vi "Create WebProxy.vi"(4 "BypassProxyOnLocal":bool, 5 "WebProxy":refnum<class "WebProxy_NET.lvclass">, 6 "UseDefaultCredentials [T]":bool, 8 "Error In":errorcluster, 10 "Port (443)":i32=443, 11 "Host":string) -> (0 "Error Out":errorcluster, 3 "WebProxy Out":refnum<class "WebProxy_NET.lvclass">)   [LabVIEW 2024, in "HttpClient_NET.lvlib" / "WebProxy_NET.lvclass"]
doc: "<b> </b> <b> </b>\nHttpClient_NET\nJustin Young - Viviota\nCopyright (c) 2021\nLicense: BSD"
uses:
  WebProxy_NET.lvclass
  WebProxy_NET.lvclass/WebProxy_NET.ctl
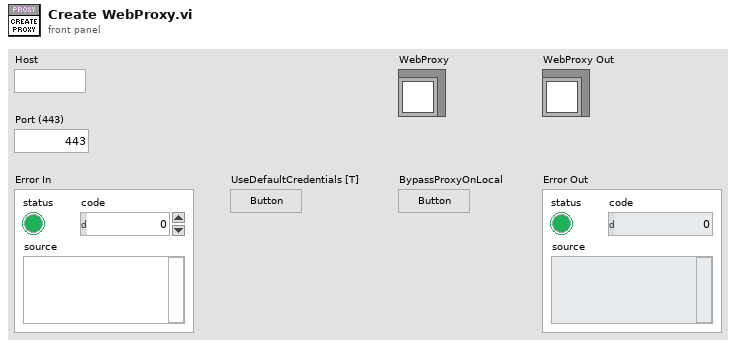
[diagram p1: front panel]
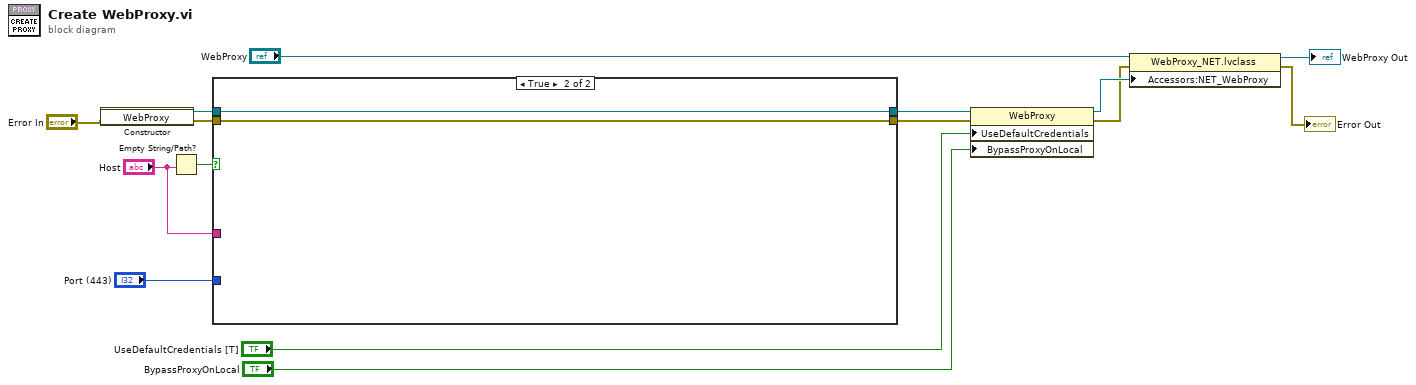
[diagram p0: block diagram]
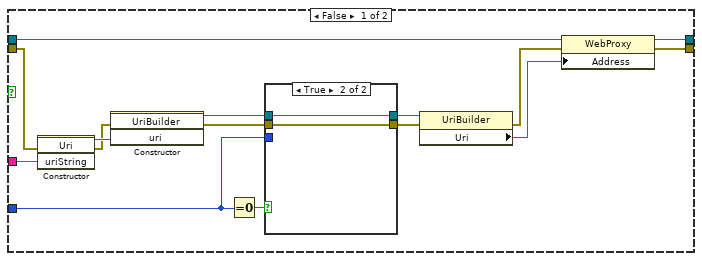
[diagram p2: hidden frame]
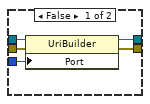
[diagram p3: hidden frame]
diagram:
  n1 = constructor class="WebProxy"(error in="Error In") -> (reference out=w8:refnum<k24>, error out=w15:errorcluster)  [unwired: 2 in, 1 out]
  n2 = Empty String/Path?(string/path="Host") -> (empty?=w4:bool)
  n3 = case shown="True" w4 {
    tunnel: w15 -> [w18 w38]
    tunnel: [w30 w38] -> w9
    tunnel: w8 -> [w29 w39]
    tunnel: [w28 w39] -> w7
    tunnel: "Host" -> [w27 _]
    tunnel: "Port (443)" -> [w26 _]
    frame False {
      n4 = constructor class="Uri"(error in=w18, "uriString"=w27) -> (reference out=w22:refnum<k24>, error out=w17:errorcluster)  [unwired: 2 in, 2 out]
      n5 = constructor class="UriBuilder"(error in=w17, "uri"=w22) -> (reference out=w23:refnum<k24>, error out=w24:errorcluster)  [unwired: 2 in, 2 out]
      n6 = Equal To 0?(x=w26) -> (x = 0?=w19:bool)
      n7 = case shown="True" w19 {
        tunnel: w24 -> [w35 w36]
        tunnel: w23 -> [w34 w37]
        tunnel: w26 -> [w33 _]
        tunnel: [w32 w37] -> w21
        tunnel: [w31 w36] -> w20
        frame False {
          n8 = property class="UriBuilder"(reference=w34, error in=w35, "Port"=w33) -> (reference out=w32:refnum<k24>, error out=w31:errorcluster)
        }
        frame True {
        }
      }
      n9 = property class="UriBuilder"(reference=w21, error in=w20) -> (error out=w16:errorcluster, "Uri"=w25:refnum<k24>)  [unwired: 1 out]
      n10 = property class="WebProxy"(reference=w29, error in=w16, "Address"=w25) -> (reference out=w28:refnum<k24>, error out=w30:errorcluster)
    }
    frame True {
    }
  }
  n11 = property class="WebProxy"(reference=w7, error in=w9, "UseDefaultCredentials"="UseDefaultCredentials [T]", "BypassProxyOnLocal"="BypassProxyOnLocal") -> (reference out=w11:refnum<k24>, error out=w3:errorcluster)
  n12 = property class="WebProxy_NET.lvclass"(reference="WebProxy", error in=w3, "Accessors:NET_WebProxy"=w11) -> (reference out=→"WebProxy Out":refnum<class "WebProxy_NET.lvclass">, error out=→"Error Out":errorcluster)
